vi "Get Unit Information.vi"(8 "error in (no error)":errorcluster, 11 "ENET_BS1200 in":refnum<class "ENET_BS1200.lvclass">) -> (0 "error out":errorcluster, 1 "Firmware":string, 2 "SerialNumber":string, 3 "ENET_BS1200 out":refnum<class "ENET_BS1200.lvclass">, 4 "Calibration Date":string)   [LabVIEW 2021, in "BS120x Driver.lvlib" / "ENET_BS1200.lvclass"]
uses:
  ENET_BS1200.lvclass
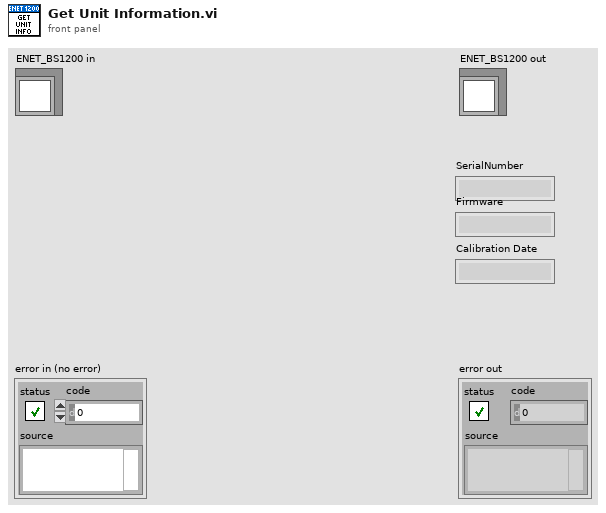
[diagram p1: front panel]
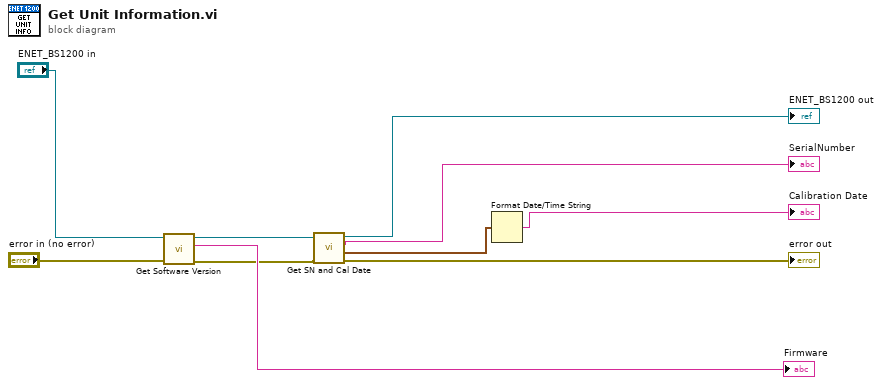
[diagram p0: block diagram]
diagram:
  n1 = call "Get Software Version.vi"("error in (no error)"="error in (no error)", "Ethernet in"="ENET_BS1200 in") -> ("error out"=w7:errorcluster, "Version"=→"Firmware":string, "Ethernet out"=w6:refnum<class "ENET_BS1200.lvclass">)  [unwired: 7 in]
  n2 = call "Get SN and Cal Date.vi"("error in (no error)"=w7, "ENET_BS1200 in"=w6) -> ("error out"=→"error out":errorcluster, "Calibration Date"=w2:timestamp, "Serial Number"=→"SerialNumber":string, "ENET_BS1200 out"=→"ENET_BS1200 out":refnum<class "ENET_BS1200.lvclass">)  [unwired: 6 in]
  n3 = Format Date/Time String(seconds (now)=w2) -> (date/time string=→"Calibration Date":string)  [unwired: 2 in]
